vi "Initialize OOB Communications.vi"(8 "error in (no error)":errorcluster, 11 "CIFTemplatePlugin in":refnum<class "TemplatePlugin.lvclass">) -> (0 "error out":errorcluster, 3 "CIFTemplatePlugin out":refnum<class "TemplatePlugin.lvclass">)   [LabVIEW 2021, in "TemplatePlugin.lvclass"]
uses:
  TemplatePlugin.lvclass
  TemplatePlugin.lvclass/TemplatePlugin.ctl
  Common/Typedef/OOB Comm/To gRPC Command Payload.ctl
  Common/Typedef/OOB Comm/To gRPC Command.ctl
  Common/Typedef/OOB Comm/To gRPC Command Data.ctl
  Common/Typedef/OOB Comm/To Main Command Payload.ctl
  Common/Typedef/OOB Comm/To Main Command.ctl
  Common/Typedef/OOB Comm/To Main Command Data.ctl
  ae490f7e-ea51-45c5-9096-bb0a4a91a057.vi
  2b7fb692-21fb-473b-8b0a-ad6086370566.vi
  339e5d9b-c057-4f7a-80d0-41b8249bc7cc.vi
  51e4a3b8-6916-4728-9df7-a3153771836c.vi
  ae490f7e-ea51-45c5-9096-bb0a4a91a057.vi/49b3dd2d-4579-4089-b72e-3f0875c862f2.vi
  <vilib>/CIF Foundation/CIF CIPC/SubVIs/Check Error.vi
  <vilib>/CIF Foundation/CIF CIPC/SubVIs/Get dll Path.vi
  2b7fb692-21fb-473b-8b0a-ad6086370566.vi/49b3dd2d-4579-4089-b72e-3f0875c862f2.vi
  339e5d9b-c057-4f7a-80d0-41b8249bc7cc.vi/49b3dd2d-4579-4089-b72e-3f0875c862f2.vi
  51e4a3b8-6916-4728-9df7-a3153771836c.vi/49b3dd2d-4579-4089-b72e-3f0875c862f2.vi
  <vilib>/Utility/error.llb/Trim Whitespace.vi
  <vilib>/string/Create NI GUID.vi
  <vilib>/CIF Foundation/CIF CIPC/SubVIs/Get Element Description Variant.vi
  <vilib>/Utility/error.llb/Error Cluster From Error Code.vi
  Common/TemplateCommon.lvlib
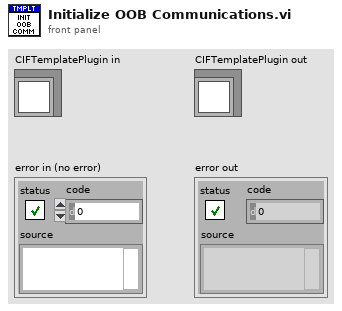
[diagram p1: front panel]
types:
  T1 = typedef "TemplateCommon.lvlib/To gRPC Command Payload.ctl" = cluster{"-> gRPC Command":T2, "-> gRPC Data":T3}
  T2 = typedef "TemplateCommon.lvlib/To gRPC Command.ctl" = enum16{"Read Data", "Read DVR Data"}
  T3 = typedef "TemplateCommon.lvlib/To gRPC Command Data.ctl" = cluster{"Cmd Data 1 -> gRPC":i32}
  T4 = typedef "TemplateCommon.lvlib/To Main Command Payload.ctl" = cluster{"Command":T5, "-> Main":T6}
  T5 = typedef "TemplateCommon.lvlib/To Main Command.ctl" = enum16{"Read Data", "Read DVR Data"}
  T6 = typedef "TemplateCommon.lvlib/To Main Command Data.ctl" = cluster{"Cmd Data 1 -> Main":i32}
  T7 = typedef "TemplateCommon.lvlib/To Main DVR Data.ctl" = cluster{"Data 1 DVR  -> Main":i32}
  T8 = typedef "TemplateCommon.lvlib/To gRPC DVR Data.ctl" = cluster{"Data 1 DVR -> gRPC ":i32}
  T9 = typedef "TemplateCommon.lvlib/To Main Cyclic Data.ctl" = cluster{"Data 1 -> Main":i32}
  T10 = typedef "TemplateCommon.lvlib/To gRPC Cyclic Data.ctl" = cluster{"Data 1 -> gRPC":i32}
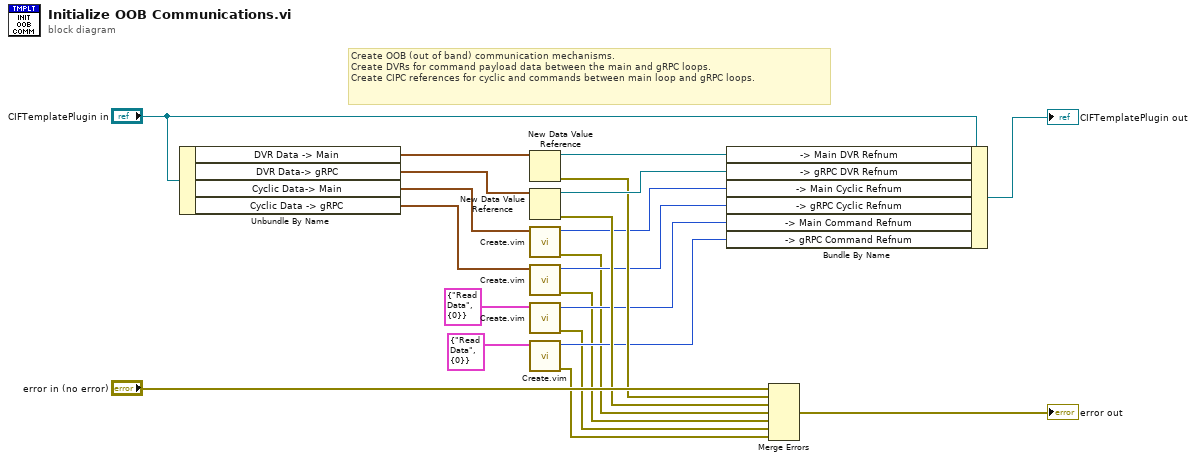
[diagram p0: block diagram]
diagram:
  # "Create OOB (out of band) communication mechanisms.\nCreate DVRs for command payload data between the main and gRPC loops. \nCreate CIPC references for cyclic and commands between main loop and gRPC loops."
  n1 = Unbundle By Name("CIFTemplatePlugin in") -> ("DVR Data -> Main"=w21:T7, "DVR Data-> gRPC"=w22:T8, "Cyclic Data-> Main"=w11:T9, "Cyclic Data -> gRPC"=w10:T10)
  n2 = New Data Value Reference(data value=w21) -> (data value reference=w18:refnum<data-value>, error out=w15:errorcluster)  [unwired: 1 in]
  n3 = New Data Value Reference(data value=w22) -> (data value reference=w17:refnum<data-value>, error out=w14:errorcluster)  [unwired: 1 in]
  n4 = call "Create.vim"("Data Type"=w11) -> ("error out"=w4:errorcluster, "CIPC Reference"=w12:u64)  [unwired: 7 in, 2 out]
  n5 = call "Create.vim"("Data Type"=w10) -> ("error out"=w3:errorcluster, "CIPC Reference"=w8:u64)  [unwired: 7 in, 2 out]
  n6 = call "Create.vim"("Data Type"=T4 {"Command"=enum."Read Data", "-> Main"={"Cmd Data 1 -> Main"=0}} ("Payload")) -> ("error out"=w2:errorcluster, "CIPC Reference"=w7:u64)  [unwired: 7 in, 2 out]
  n7 = call "Create.vim"("Data Type"=T1 {"-> gRPC Command"=enum."Read Data", "-> gRPC Data"={"Cmd Data 1 -> gRPC"=0}} ("-> gRPC Payload")) -> ("error out"=w1:errorcluster, "CIPC Reference"=w5:u64)  [unwired: 7 in, 2 out]
  n8 = Bundle By Name(cluster="CIFTemplatePlugin in", "-> Main DVR Refnum"=w18, "-> gRPC DVR Refnum"=w17, "-> Main Cyclic Refnum"=w12, "-> gRPC Cyclic Refnum"=w8, "-> Main Command Refnum"=w7, "-> gRPC Command Refnum"=w5) -> (→"CIFTemplatePlugin out":refnum<class "TemplatePlugin.lvclass">)
  n9 = Merge Errors("error in (no error)", w15, w14, w4, w3, w2, w1) -> (→"error out":errorcluster)
